vi "emi_Num U8 to BCD U8.vi"(7 "Numeric":u8) -> (8 "BCD":u8, 10 "Valid Numeric BCD":bool)   [LabVIEW 2010]
doc: "Numeric must have a vlaue 0 and 99, if it is heigher the Valid Numeric BCD flag will NOT be set, and the contents of BCD is uncertain. \n\nResult will be a BCD value with value between '0''0' and '9''9' (if valid).\ns"
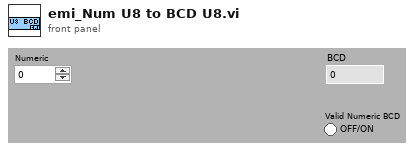
[diagram p1: front panel]
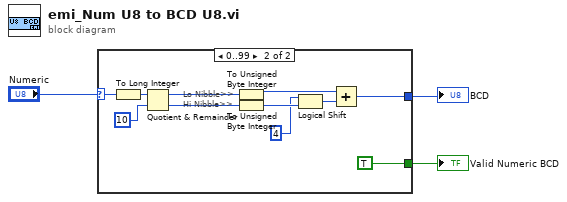
[diagram p0: block diagram]
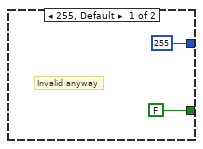
[diagram p2: hidden frame]
diagram:
  n1 = case shown="0..99" "Numeric" {
    selector: "Numeric" -> [_ w6]
    tunnel: [u8 255 w7] -> w3
    tunnel: [FALSE TRUE] -> w2
    frame 255, Default {
      # "Invalid anyway"
    }
    frame 0..99 {
      # "Hi Nibble>>"
      # "Lo Nibble>>"
      n2 = To Long Integer(number=w6) -> (32bit integer=w14:i32)
      n3 = Quotient & Remainder(x=w14, y=10) -> (x-y*floor(x/y)=w13:i32, floor(x/y)=w12:i32)
      n4 = To Unsigned Byte Integer(number=w13) -> (unsigned 8bit integer=w8:u8)
      n5 = To Unsigned Byte Integer(number=w12) -> (unsigned 8bit integer=w11:u8)
      n6 = Logical Shift(y=i8 4, x=w11) -> (x << y=w9:u8)
      n7 = Add(x=w8, y=w9) -> (x+y=w7:u8)
    }
  }
  "BCD" <- w3
  "Valid Numeric BCD" <- w2
